vi "FlowPID3.vi"() -> ()   [LabVIEW 2017]
uses:
  BERTTA.dll
panel:
  out "Setpoint RPM":dbl
  out "lastWeight":dbl
  in  "Setpoint_W":dbl=25.0
  in  "port_mettler":i32=35
  in  "port_isma":i32=38
  out "lasttime":dbl
  out "timechange":dbl
  out "error":dbl
  out "errsum":dbl
  out "output2":dbl
  out "Waveform Chart":dynamicdata(graph)
  in  "kd":dbl
  in  "ki":dbl=1e-05
  in  "kp":dbl=0.001
  in  "Setpoint_T":dbl=5.0
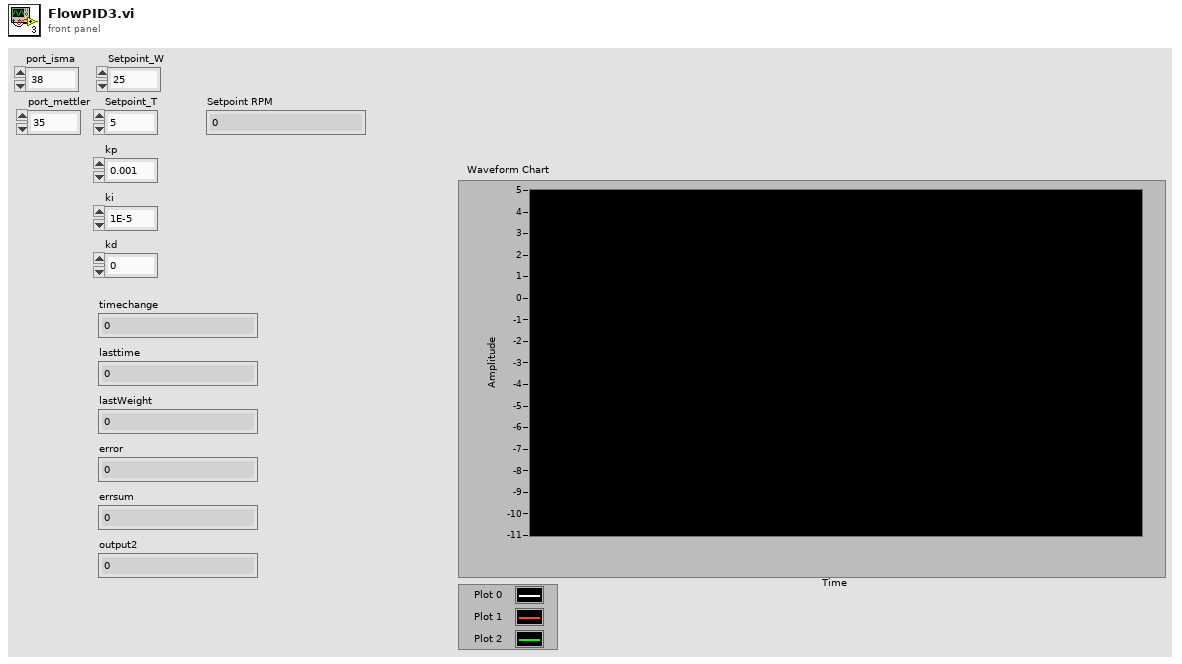
[diagram p1: front panel]
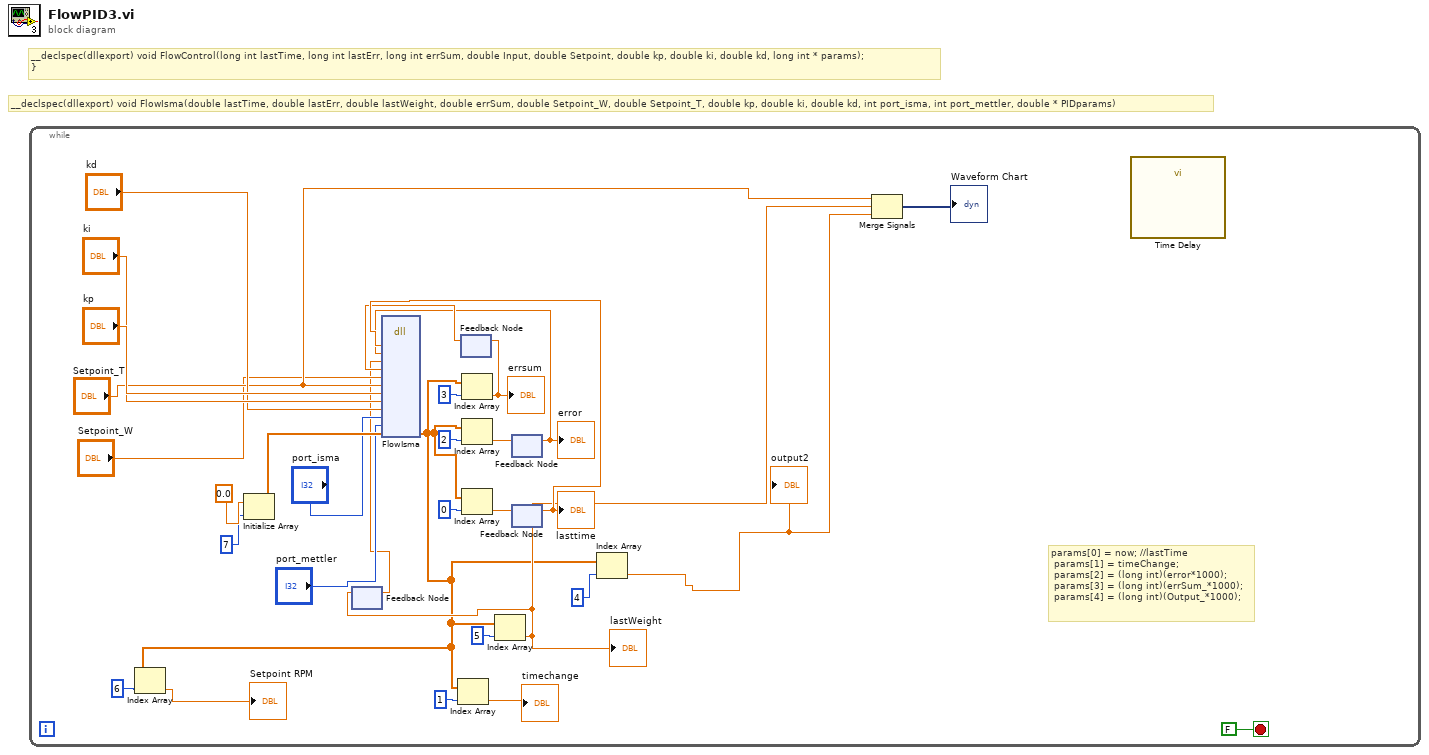
[diagram p0: block diagram]
diagram:
  # "__declspec(dllexport) void FlowIsma(double lastTime, double lastErr, double lastWeight, double errSum, double Setpoint_W, double Setpoint_T, double kp, double ki, double kd, int port_isma, int port_mettler, double * PIDparams)"
  # "__declspec(dllexport) void FlowControl(long int lastTime, long int lastErr, long int errSum, double Input, double Setpoint, double kp, double ki, double kd, long int * params);\n}"
  n1 = while {
    stop <- FALSE stop-if-true
    # "params[0] = now; //lastTime\n\tparams[1] = timeChange;\n\tparams[2] = (long int)(error*1000);\n\tparams[3] = (long int)(errSum_*1000);\n\tparams[4] = (long int)(Output_*1000);"
    n2 = Initialize Array(0.0 ("element"), 7 ("dimension size")) -> (w28:dbl[])
    n3 = feedback #1() -> (w5:dbl)  [unwired: 1 in]
    n4 = feedback #2() -> (w15:dbl)  [unwired: 1 in]
    n5 = feedback #3() -> (w11:dbl)  [unwired: 1 in]
    "error" <- w11
    n6 = feedback #4() -> (w21:dbl)  [unwired: 1 in]
    "lasttime" <- w21
    n7 = dll-call lib="C:/Users/p3cn/OneDrive - Kemira Oyj/Documents/GitHub/Bertta/BERTTA/x64/Release/BERTTA.dll" fn="FlowIsma"("lastTime"=w21, "lastErr"=w11, "lastWeight"=w5, "errSum"=w15, "Setpoint_W"="Setpoint_W", "Setpoint_T"="Setpoint_T", "kp"="kp", "ki"="ki", "kd"="kd", "port_isma"="port_isma", "port_mettler"="port_mettler", "PIDparams"=w28) -> ("PIDparams"=w2:dbl[])  [unwired: 15 in, 2 out]
    n8 = Index Array(array=w2, index=6) -> (element=→"Setpoint RPM":dbl)
    n9 = Index Array(array=w2, index=1) -> (element=→"timechange":dbl)
    n10 = Index Array(array=w2, index=3) -> (element=w16:dbl)
    "errsum" <- w16
    n11 = feedback-in #2(w16) -> ()
    n12 = Index Array(array=w2, index=2) -> (element=w18:dbl)
    n13 = Index Array(array=w2, index=0) -> (element=w22:dbl)
    n14 = Index Array(array=w2, index=5) -> (element=w4:dbl)
    "lastWeight" <- w4
    n15 = feedback-in #1(w4) -> ()
    n16 = feedback-in #3(w18) -> ()
    n17 = feedback-in #4(w22) -> ()
    n18 = Index Array(array=w2, index=4) -> (element=w10:dbl)
    "output2" <- w10
    n19 = Merge Signals("Setpoint_T", w4, w10) -> (→"Waveform Chart":dynamicdata)
    n20 = call "Time Delay"() -> ()  [unwired: 11 in, 1 out]
  }
